vi "ExSubSnapNStore.vi"(2 "error in (no error)":errorcluster, 3 "Handle Cluster":T1) -> (0 "error out":errorcluster, 1 "Handle Cluster Out":T1)   [LabVIEW 2010]
panel:
  # "ExSubSnapNStore: this VI\nStarts the camera and collects\none image and stores it.\nNote the camera should be in \nAsync mode for this sub vi"
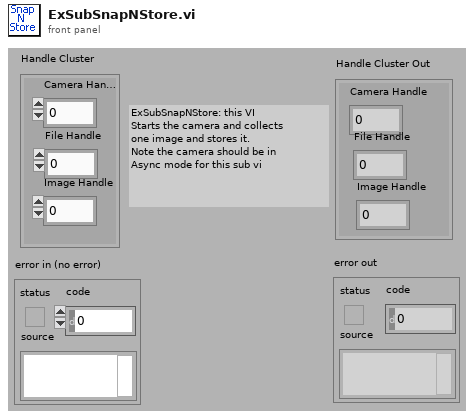
[diagram p1: front panel]
types:
  T1 = cluster{"Camera Handle":u32, "File Handle":u32, "Image Handle":u32}
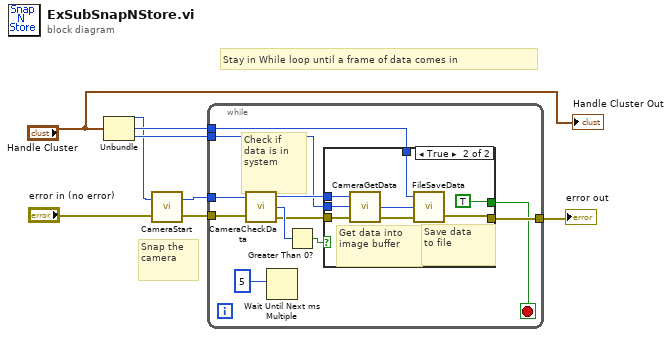
[diagram p0: block diagram]
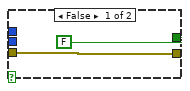
[diagram p2: hidden frame]
diagram:
  # "Snap the\ncamera"
  # "Stay in While loop until a frame of data comes in"
  n1 = Unbundle("Handle Cluster") -> ("Camera Handle"=w5:u32, "File Handle"=w7:u32, "Image Handle"=w6:u32)
  n2 = call <userlib>:"CameraStart.vi"("error in"="error in (no error)", "Camera Handle"=w5) -> ("error out"=w3:errorcluster, "Camera Handle"=w2:u32)
  n3 = while {
    tunnel: w3 -> [w15]
    tunnel: [w14] -> w8
    tunnel: w7 -> [w13]
    tunnel: w6 -> [w12]
    tunnel: w2 -> [w10]
    stop <- w11 stop-if-true
    # "Check if \ndata is in\nsystem"
    n4 = call <userlib>:"CameraCheckData.vi"("Camera Handle"=w10, "error in"=w15) -> ("Camera Handle"=w18:u32, "Number Of Frames Available"=w17:i32, "error out"=w16:errorcluster)
    n5 = Wait Until Next ms Multiple(millisecond multiple=5) -> ()  [unwired: 1 out]
    n6 = Greater Than 0?(x=w17) -> (x > 0?=w19:bool)
    n7 = case shown="True" w19 {
      tunnel: w18 -> [_ w29]
      tunnel: w16 -> [w21 w28]
      tunnel: [w21 w24] -> w14
      tunnel: [FALSE TRUE] -> w11
      tunnel: w13 -> [_ w23]
      tunnel: w12 -> [_ w22]
      frame False {
      }
      frame True {
        # "Save data \nto file"
        # "Get data into\nimage buffer"
        n8 = call <userlib>:"CameraGetData.vi"("error in"=w28, "Data Handle"=w22, "Camera Handle"=w29) -> ("error out"=w27:errorcluster, "Data Handle"=w26:u32)  [unwired: 1 out]
        n9 = call <userlib>:"FileSaveData.vi"("error in"=w27, "Image Handle"=w26, "File Handle"=w23) -> ("error out"=w24:errorcluster)  [unwired: 1 out]
      }
    }
  }
  "error out" <- w8
  "Handle Cluster Out" <- "Handle Cluster"
